vi "注销.vi"(8 "error in (no error)":errorcluster caption="错误输入（无错误）", 10 "数据值引用":refnum<data-value>, 11 "数据采集 输入":refnum<class "数据采集.lvclass"> caption="DNL_LabVIEW Object in") -> (0 "error out":errorcluster caption="错误输出", 3 "数据采集 输出":refnum<class "数据采集.lvclass"> caption="DNL_LabVIEW Object out")   [LabVIEW 2013, in "数据采集.lvclass"]
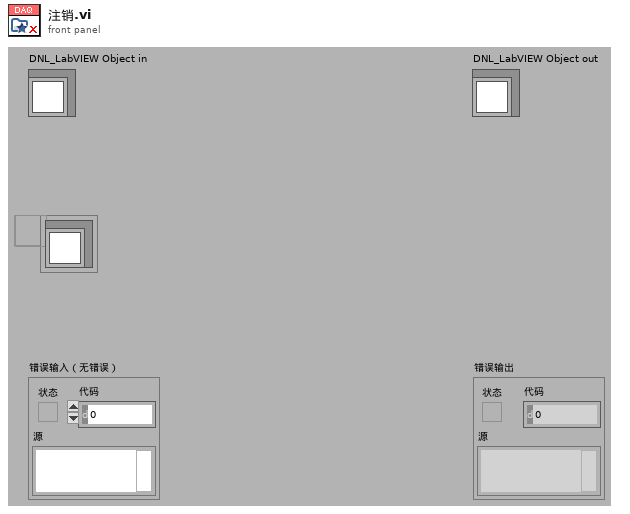
[diagram p1: front panel]
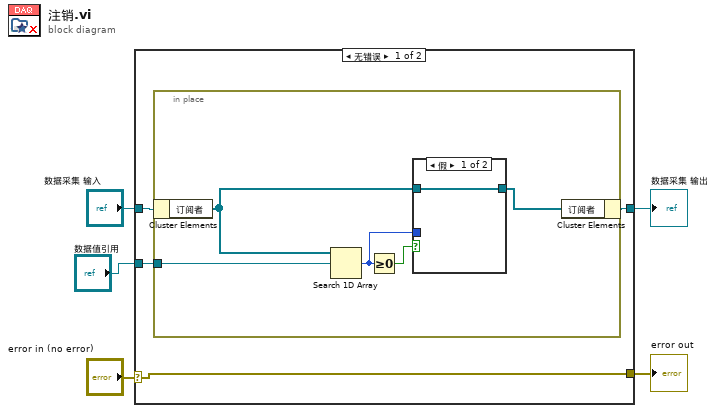
[diagram p0: block diagram]
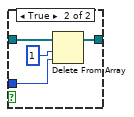
[diagram p2: hidden frame]
diagram:
  n1 = case shown="无错误" "error in (no error)" {
    selector: "error in (no error)" -> [w6 w21]
    tunnel: [w6 w21] -> w4
    tunnel: [w8 w20] -> w2
    tunnel: "数据采集 输入" -> [w9 w20]
    tunnel: "数据值引用" -> [w7 _]
    frame No Error {
      n2 = in-place {
        in-place-border: w7 -> [w12]
        n3 = in-place-cluster #1(w9) -> ("订阅者"=w11:refnum<data-value>[])
        n4 = Search 1D Array(1D array=w11, element=w12) -> (index of element=w13:i32)  [unwired: 1 in]
        n5 = Greater Or Equal To 0?(x=w13) -> (x >= 0?=w14:bool)
        n6 = case shown="假" w14 {
          tunnel: w13 -> [_ w18]
          tunnel: [w15 w17] -> w10
          tunnel: w11 -> [w15 w16]
          frame False {
          }
          frame True {
            n7 = Delete From Array(array=w16, length=1 ("长度"), index=w18) -> (array with subset deleted=w17:refnum<data-value>[])  [unwired: 1 out]
          }
        }
        n8 = in-place-cluster #1("订阅者"=w10) -> (w8:refnum<class "数据采集.lvclass">)
      }
    }
    frame Error {
    }
  }
  "error out" <- w4
  "数据采集 输出" <- w2
